vi "ConvertVoltageToPercentVbs.vi"(11 "Voltage":dbl) -> (3 "Vbus":dbl)   [LabVIEW 2015]
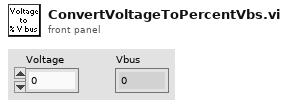
[diagram p1: front panel]
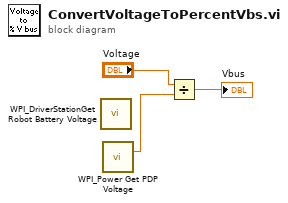
[diagram p0: block diagram]
diagram:
  n1 = call <vilib>:"WPI_DriverStationGet Robot Battery Voltage.vi"() -> ()  [unwired: 14 in, 2 out]
  n2 = call <vilib>:"WPI_Power Get PDP Voltage.vi"() -> ("voltage (V)"=w1:dbl)  [unwired: 14 in, 1 out]
  n3 = Divide(x="Voltage", y=w1) -> (x/y=→"Vbus":dbl)
